vi "hse-application_SelectProjectFolder.vi"(8 "error in":errorcluster, 10 "Start path":path) -> (0 "error out":errorcluster, 2 "PROJECT Folder":path, 3 "PROJECT Name":string)   [LabVIEW 2014, in "hse-application.lvclass"]
doc: "Opens a file dialog to select the folder in which the project file and the startup.vi are located.\n\n____\nHAMPEL SOFTWARE ENGINEERING v0.12.0 (2018-09-13 18:21)"
uses:
  hse-application.lvclass
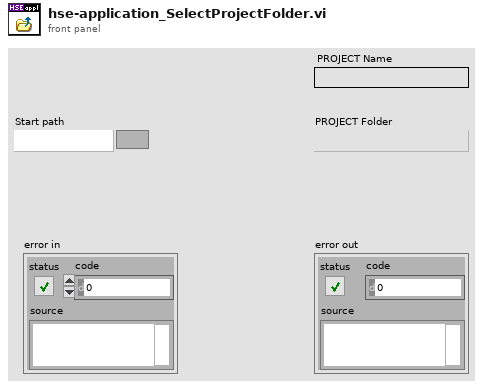
[diagram p1: front panel]
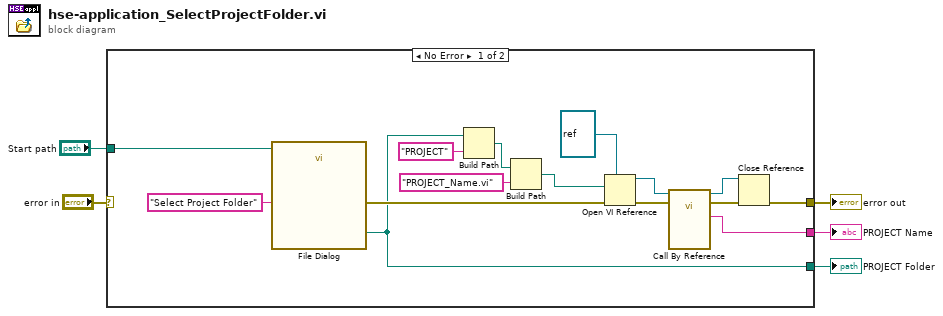
[diagram p0: block diagram]
diagram:
  n1 = case shown="No Error" "error in" {
    selector: "error in" -> [_ w21]
    tunnel: [w20 _] -> w5
    tunnel: "Start path" -> [w12 _]
    tunnel: [w9 w21] -> w3
    tunnel: [w8 _] -> w2
    frame No Error {
      n2 = call "File Dialog"("start path"=w12, "prompt"="Select Project Folder") -> ("selected path"=w8:path, "error out"=w19:errorcluster)  [unwired: 10 in, 2 out]
      n3 = Build Path(base path=w8, name or relative path="PROJECT") -> (appended path=w14:path)
      n4 = Build Path(base path=w14, name or relative path="PROJECT_Name.vi") -> (appended path=w6:path)
      n5 = Open VI Reference(type specifier VI Refnum (for type only)=refnum<vi> refnum, vi path=w6, error in (no error)=w19) -> (vi reference=w16:refnum<vi>, error out=w17:errorcluster)  [unwired: 3 in]
      n6 = call-by-ref "?"(reference=w16, error in=w17) -> (reference out=w10:refnum<vi>, error out=w11:errorcluster, "PROJECT Name"=w20:string)  [unwired: 11 in]
      n7 = Close Reference(reference=w10, error in (no error)=w11) -> (error out=w9:errorcluster)
    }
    frame Error {
    }
  }
  "PROJECT Folder" <- w2
  "PROJECT Name" <- w5
  "error out" <- w3
